vi "Get State.vi"(8 "error in":errorcluster, 9 "timeout (-1)":i32=-1, 11 "Standard Engine Runtime in":refnum<class "synchronous engine runtime.lvclass">) -> (0 "error out":errorcluster, 2 "Engine State":T1, 3 "Standard Engine Runtime out":refnum<class "synchronous engine runtime.lvclass">)   [LabVIEW 2014, in "synchronous engine runtime.lvclass"]
uses:
  synchronous engine runtime.lvclass
  Engine Runtime/Execution States.ctl
  synchronous engine runtime.lvclass/synchronous engine runtime.ctl
  Engine Runtime/Engine Runtime Interface.lvclass
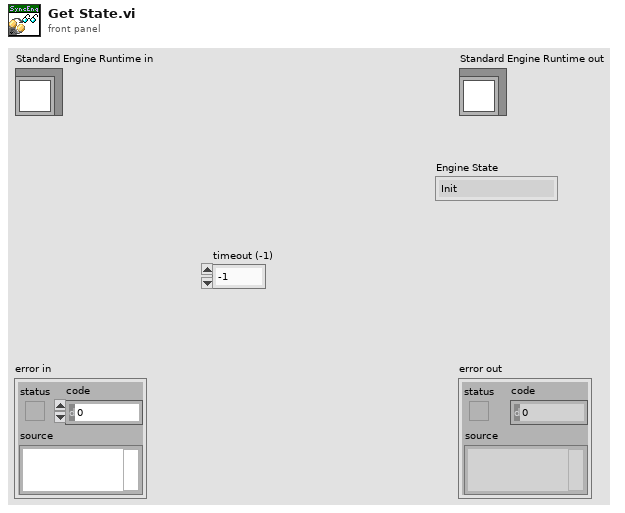
[diagram p1: front panel]
types:
  T1 = typedef "Engine Runtime Interface.lvclass/Execution States.ctl" = enum16{"Init", "Pre-Operational", "Safe-Operational", "Operational", "Stopped"}
  T2 = typedef "synchronous engine runtime.lvclass/notifier.ctl" = cluster{"Engine State":T1, "error constant":errorcluster}
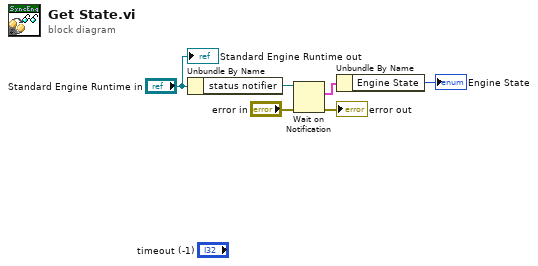
[diagram p0: block diagram]
diagram:
  n1 = Unbundle By Name("Standard Engine Runtime in") -> ("status notifier"=w5:refnum<notifier>)
  n2 = Wait on Notification(notifier=w5, error in (no error)="error in") -> (notification=w2:T2, error out=→"error out":errorcluster)  [unwired: 2 in, 2 out]
  n3 = Unbundle By Name(w2) -> ("Engine State"=→"Engine State":T1)
  "Standard Engine Runtime out" <- "Standard Engine Runtime in"
